vi "py.create.Pitch.vi"(8 "error in (no error)":errorcluster, 11 "Parameters":variant) -> (0 "error out":errorcluster, 3 "bytes":u8[](array[numeric]) format="%.0x")   [LabVIEW 2020]
uses:
  AddOrder/AddOrderLong.Parameters.ctl
  Time/Time.Parameters.ctl
  OrderExecuted/OrderExecuted.Parameters.ctl
  ReduceSize/ReduceSizeLong.Parameters.ctl
  ReduceSize/ReduceSizeShort.Parameters.ctl
  ModifyOrder/ModifyOrderLong.Parameters.ctl
  ModifyOrder/ModifyOrderShort.Parameters.ctl
  DeleteOrder/DeleteOrder.Parameters.ctl
  Trade/TradeLong.Parameters.ctl
  Trade/TradeShort.Parameters.ctl
  Trade/TradeExpanded.Parameters.ctl
  AddOrder/AddOrderShort.Parameters.ctl
  AddOrder/AddOrderExpanded.Parameters.ctl
  OrderExecuted/OrderExecutedAtPriceSize.Parameters.ctl
  <vilib>/Utility/Data Type/NI_Data Type.lvlib
  AddOrder/AddOrderLong.lvclass
  Time/Time.lvclass
  OrderExecuted/OrderExecuted.lvclass
  ReduceSize/ReduceSizeLong.lvclass
  ReduceSize/ReduceSizeShort.lvclass
  ModifyOrder/ModifyOrderLong.lvclass
  ModifyOrder/ModifyOrderShort.lvclass
  DeleteOrder/DeleteOrder.lvclass
  Trade/TradeLong.lvclass
  Trade/TradeShort.lvclass
  Trade/TradeExpanded.lvclass
  AddOrder/AddOrderShort.lvclass
  AddOrder/AddOrderExpanded.lvclass
  OrderExecuted/OrderExecutedAtPriceSize.lvclass
panel:
  out "return value":string
  out "Application Directory":path
  out "name":string
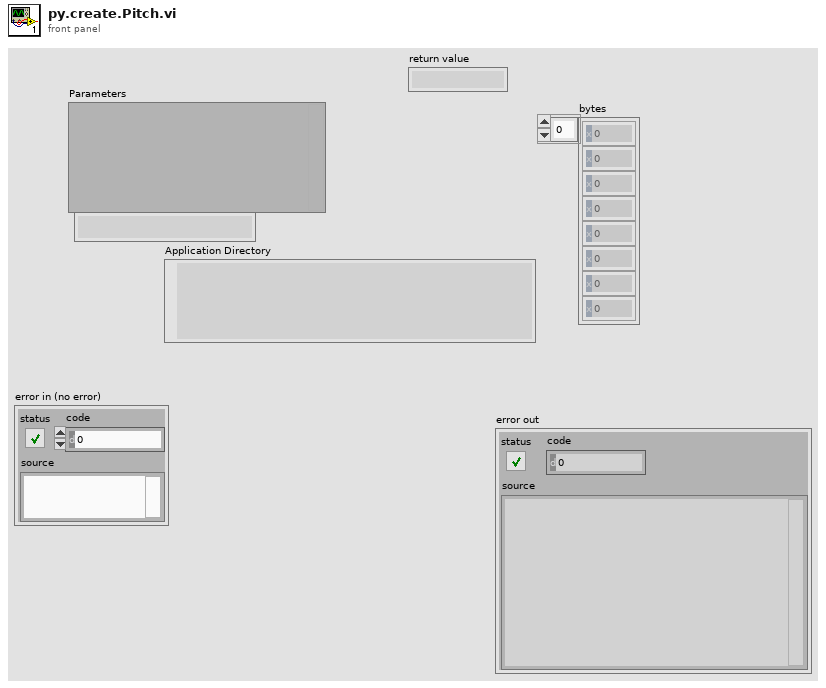
[diagram p1: front panel]
types:
  T1 = typedef "AddOrderLong.lvclass/AddOrderLong.Parameters.ctl" = cluster{"Time Offset":u32, "Order Id":string, "Quantity":u32, "Symbol":string, "Side Indicator":string, "Price":dbl}
  T2 = typedef "Time.lvclass/Time.Parameters.ctl" = cluster{"Time":u32}
  T3 = typedef "OrderExecuted.lvclass/OrderExecuted.Parameters.ctl" = cluster{"Time Offset":u32, "Order Id":string, "Executed Quantity":u32, "Execution Id":string}
  T4 = typedef "ReduceSizeLong.lvclass/ReduceSizeLong.Parameters.ctl" = cluster{"Time Offset":u32, "Order Id":string, "Canceled Quantity":u32}
  T5 = typedef "ReduceSizeShort.lvclass/ReduceSizeShort.Parameters.ctl" = cluster{"Time Offset":u32, "Order Id":string, "Canceled Quantity":u16}
  T6 = typedef "ModifyOrderLong.lvclass/ModifyOrderLong.Parameters.ctl" = cluster{"Time Offset":u32, "Order Id":string, "Quantity":u32, "Price":dbl, "Modify Flags":u8}
  T7 = typedef "ModifyOrderShort.lvclass/ModifyOrderShort.Parameters.ctl" = cluster{"Time Offset":u32, "Order Id":string, "Quantity":u32, "Price":u16, "Modify Flags":u8}
  T8 = typedef "DeleteOrder.lvclass/DeleteOrder.Parameters.ctl" = cluster{"Time Offset":u32, "Order Id":string}
  T9 = typedef "TradeLong.lvclass/TradeLong.Parameters.ctl" = cluster{"Time Offset":u32, "Order Id":string, "Execution Id":string, "Quantity":u32, "Price":dbl, "Side Indicator":string, "Symbol":string}
  T10 = typedef "TradeShort.lvclass/TradeShort.Parameters.ctl" = cluster{"Time Offset":u32, "Order Id":string, "Execution Id":string, "Quantity":u32, "Price":dbl, "Side Indicator":string, "Symbol":string}
  T11 = typedef "TradeExpanded.lvclass/TradeExpanded.Parameters.ctl" = cluster{"Time Offset":u32, "Order Id":string, "Side Indicator":string, "Quantity":u32, "Symbol":string, "Price":dbl, "Execution Id":string}
  T12 = typedef "AddOrderShort.lvclass/AddOrderShort.Parameters.ctl" = cluster{"Time Offset":u32, "Order Id":string, "Quantity":u32, "Symbol":string, "Side Indicator":string, "Price":dbl}
  T13 = typedef "AddOrderExpanded.lvclass/AddOrderExpanded.Parameters.ctl" = cluster{"Time Offset":u32, "Order Id":string, "Quantity":u32, "Symbol":string, "Side Indicator":string, "Price":dbl, "Participant Id":string, "Customer Indicator":string}
  T14 = typedef "OrderExecutedAtPriceSize.lvclass/OrderExecutedAtPriceSize.Parameters.ctl" = cluster{"Time Offset":u32, "Order Id":string, "Executed Quantity":u32, "Execution Id":string, "Remaining Quantity":u32, "Price":dbl}
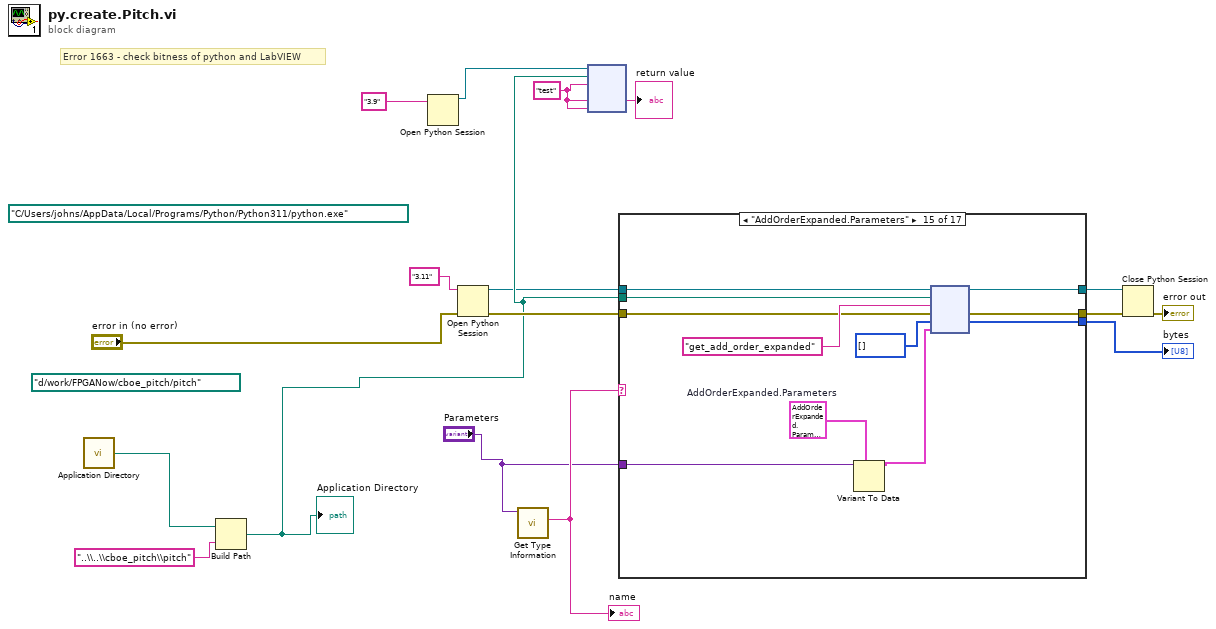
[diagram p0: block diagram]
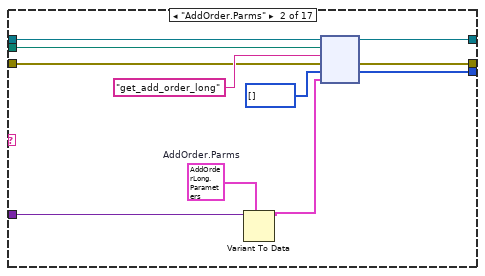
[diagram p3: hidden frame]
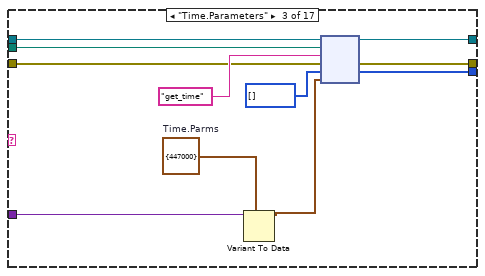
[diagram p4: hidden frame]
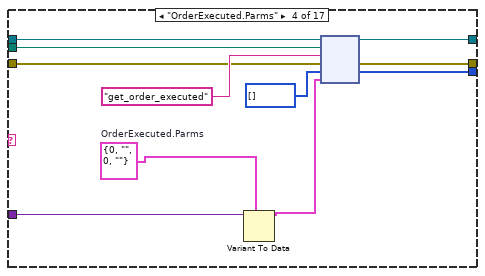
[diagram p5: hidden frame]
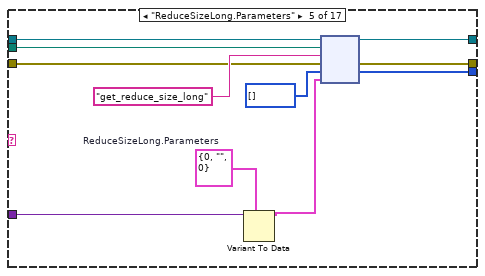
[diagram p6: hidden frame]
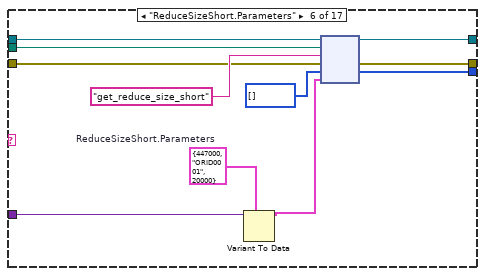
[diagram p7: hidden frame]
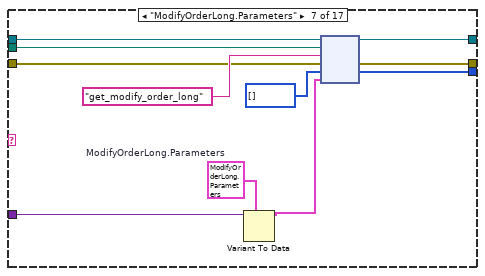
[diagram p8: hidden frame]
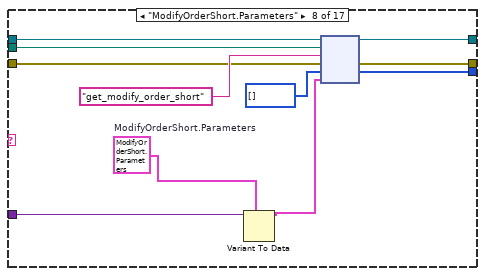
[diagram p9: hidden frame]
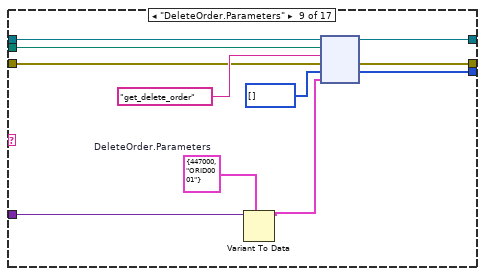
[diagram p10: hidden frame]
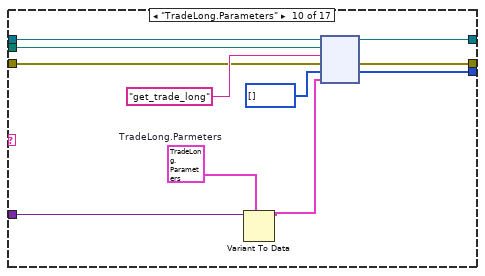
[diagram p11: hidden frame]
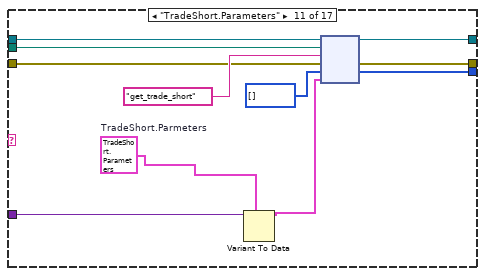
[diagram p12: hidden frame]
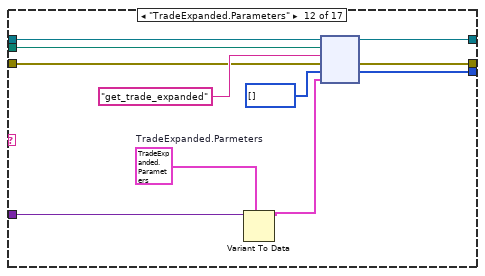
[diagram p13: hidden frame]
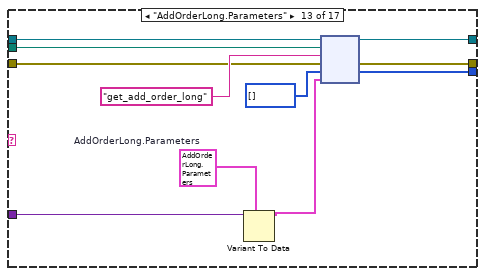
[diagram p14: hidden frame]
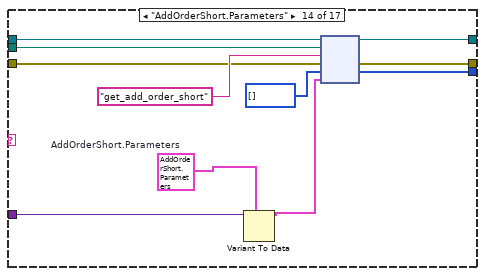
[diagram p15: hidden frame]
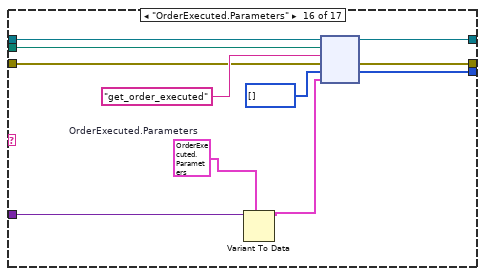
[diagram p16: hidden frame]
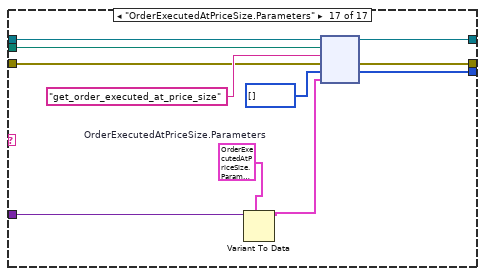
[diagram p17: hidden frame]
diagram:
  w3 = "test" ("function name")
  (unwired) path "C:/Users/johns/AppData/Local/Programs/Python/Python311/python.exe" ("Python path")
  (unwired) path "d:/work/FPGANow/cboe_pitch/pitch" ("module path")
  # "Error 1663 - check bitness of python and LabVIEW"
  n1 = call <vilib>:"Application Directory.vi"() -> ("Application Directory"=w8:path)
  n2 = Build Path(base path=w8, name or relative path="..\\..\\cboe_pitch\\pitch") -> (appended path=w6:path)
  "Application Directory" <- w6
  n3 = Open Python Session(python version="3.9" ("Python version")) -> (session out=w1:refnum<k35>)  [unwired: 2 in, 1 out]
  n4 = Open Python Session(python version="3.11" ("Python version"), 3:"error in (no error)") -> (session out=w5:refnum<k35>, error out=w14:errorcluster)  [unwired: 1 in]
  n5 = call <vilib>:"Get Type Information.vi"("variant"="Parameters") -> ("name"=w10:string)  [unwired: 6 in, 4 out]
  "name" <- w10
  n6 = node(w1, w6, w3, w3, w3) -> (→"return value":string)  [unwired: 2 in, 4 out]
  n7 = case shown="\"AddOrderExpanded.Parameters\"" w10 {
    tunnel: w5 -> [w19 w30 w41 w52 w63 w74 w85 w96 w107 w118 w129 w140 w151 w162 w173 w184 w195]
    tunnel: [w19 w29 w40 w51 w62 w73 w84 w95 w106 w117 w128 w139 w150 w161 w172 w183 w194] -> w17
    tunnel: w6 -> [_ w28 w39 w50 w61 w72 w83 w94 w105 w116 w127 w138 w149 w160 w171 w182 w193]
    tunnel: [w18 w27 w38 w49 w60 w71 w82 w93 w104 w115 w126 w137 w148 w159 w170 w181 w192] -> w15
    tunnel: w14 -> [w18 w25 w36 w47 w58 w69 w80 w91 w102 w113 w124 w135 w146 w157 w168 w179 w190]
    tunnel: [_ w24 w35 w46 w57 w68 w79 w90 w101 w112 w123 w134 w145 w156 w167 w178 w189] -> w13
    tunnel: "Parameters" -> [_ w22 w33 w44 w55 w66 w77 w88 w99 w110 w121 w132 w143 w154 w165 w176 w187]
    frame "False", Default {
    }
    frame "AddOrder.Parms" {
      w21 = T1 {"Time Offset"=447000, "Order Id"="ORID0001", "Quantity"=20000, "Symbol"="AAPL", "Side Indicator"="B", "Price"=0.905}  # AddOrder.Parms
      n8 = Variant To Data(type=w21, Variant=w22) -> (data=w20:T1)  [unwired: 1 in, 1 out]
      n9 = node(w30, w28, "get_add_order_long" ("function name"), w25, u8[] [], w20) -> (w29:refnum<k35>, w27:errorcluster, w24:u8[])  [unwired: 1 in, 2 out]
    }
    frame "Time.Parameters" {
      w31 = T2 {"Time"=447000}  # Time.Parms
      n10 = Variant To Data(type=w31, Variant=w33) -> (data=w32:T2)  [unwired: 1 in, 1 out]
      n11 = node(w41, w39, "get_time" ("function name"), w36, u8[] [], w32) -> (w40:refnum<k35>, w38:errorcluster, w35:u8[])  [unwired: 1 in, 2 out]
    }
    frame "OrderExecuted.Parms" {
      w42 = T3 {"Time Offset"=0, "Order Id"="", "Executed Quantity"=0, "Execution Id"=""}  # OrderExecuted.Parms
      n12 = Variant To Data(type=w42, Variant=w44) -> (data=w43:T3)  [unwired: 1 in, 1 out]
      n13 = node(w52, w50, "get_order_executed" ("function name"), w47, u8[] [], w43) -> (w51:refnum<k35>, w49:errorcluster, w46:u8[])  [unwired: 1 in, 2 out]
    }
    frame "ReduceSizeLong.Parameters" {
      w53 = T4 {"Time Offset"=0, "Order Id"="", "Canceled Quantity"=0}  # ReduceSizeLong.Parameters
      n14 = Variant To Data(type=w53, Variant=w55) -> (data=w54:T4)  [unwired: 1 in, 1 out]
      n15 = node(w63, w61, "get_reduce_size_long" ("function name"), w58, u8[] [], w54) -> (w62:refnum<k35>, w60:errorcluster, w57:u8[])  [unwired: 1 in, 2 out]
    }
    frame "ReduceSizeShort.Parameters" {
      w64 = T5 {"Time Offset"=447000, "Order Id"="ORID0001", "Canceled Quantity"=20000}  # ReduceSizeShort.Parameters
      n16 = Variant To Data(type=w64, Variant=w66) -> (data=w65:T5)  [unwired: 1 in, 1 out]
      n17 = node(w74, w72, "get_reduce_size_short" ("function name"), w69, u8[] [], w65) -> (w73:refnum<k35>, w71:errorcluster, w68:u8[])  [unwired: 1 in, 2 out]
    }
    frame "ModifyOrderLong.Parameters" {
      w75 = T6 {"Time Offset"=447000, "Order Id"="ORID0001", "Quantity"=20000, "Price"=0.905, "Modify Flags"=1}  # ModifyOrderLong.Parameters
      n18 = Variant To Data(type=w75, Variant=w77) -> (data=w76:T6)  [unwired: 1 in, 1 out]
      n19 = node(w85, w83, "get_modify_order_long" ("function name"), w80, u8[] [], w76) -> (w84:refnum<k35>, w82:errorcluster, w79:u8[])  [unwired: 1 in, 2 out]
    }
    frame "ModifyOrderShort.Parameters" {
      w86 = T7 {"Time Offset"=447000, "Order Id"="ORID0001", "Quantity"=20000, "Price"=1, "Modify Flags"=1}  # ModifyOrderShort.Parameters
      n20 = Variant To Data(type=w86, Variant=w88) -> (data=w87:T7)  [unwired: 1 in, 1 out]
      n21 = node(w96, w94, "get_modify_order_short" ("function name"), w91, u8[] [], w87) -> (w95:refnum<k35>, w93:errorcluster, w90:u8[])  [unwired: 1 in, 2 out]
    }
    frame "DeleteOrder.Parameters" {
      w97 = T8 {"Time Offset"=447000, "Order Id"="ORID0001"}  # DeleteOrder.Parameters
      n22 = Variant To Data(type=w97, Variant=w99) -> (data=w98:T8)  [unwired: 1 in, 1 out]
      n23 = node(w107, w105, "get_delete_order" ("function name"), w102, u8[] [], w98) -> (w106:refnum<k35>, w104:errorcluster, w101:u8[])  [unwired: 1 in, 2 out]
    }
    frame "TradeLong.Parameters" {
      w108 = T9 {"Time Offset"=447000, "Order Id"="ORID0001", "Execution Id"="EXE_ID_1", "Quantity"=20000, "Price"=0.905, "Side Indicator"="B", "Symbol"="AAPL"}  # TradeLong.Parmeters
      n24 = Variant To Data(type=w108, Variant=w110) -> (data=w109:T9)  [unwired: 1 in, 1 out]
      n25 = node(w118, w116, "get_trade_long" ("function name"), w113, u8[] [], w109) -> (w117:refnum<k35>, w115:errorcluster, w112:u8[])  [unwired: 1 in, 2 out]
    }
    frame "TradeShort.Parameters" {
      w119 = T10 {"Time Offset"=447000, "Order Id"="ORID0001", "Execution Id"="EXE_ID_1", "Quantity"=20000, "Price"=0.905, "Side Indicator"="B", "Symbol"="AAPL"}  # TradeShort.Parmeters
      n26 = Variant To Data(type=w119, Variant=w121) -> (data=w120:T10)  [unwired: 1 in, 1 out]
      n27 = node(w129, w127, "get_trade_short" ("function name"), w124, u8[] [], w120) -> (w128:refnum<k35>, w126:errorcluster, w123:u8[])  [unwired: 1 in, 2 out]
    }
    frame "TradeExpanded.Parameters" {
      w130 = T11 {"Time Offset"=447000, "Order Id"="ORID0001", "Side Indicator"="B", "Quantity"=20000, "Symbol"="AAPL", "Price"=0.905, "Execution Id"="EXE_ID_1"}  # TradeExpanded.Parmeters
      n28 = Variant To Data(type=w130, Variant=w132) -> (data=w131:T11)  [unwired: 1 in, 1 out]
      n29 = node(w140, w138, "get_trade_expanded" ("function name"), w135, u8[] [], w131) -> (w139:refnum<k35>, w137:errorcluster, w134:u8[])  [unwired: 1 in, 2 out]
    }
    frame "AddOrderLong.Parameters" {
      w141 = T1 {"Time Offset"=447000, "Order Id"="ORID0001", "Quantity"=20000, "Symbol"="AAPL", "Side Indicator"="B", "Price"=0.905}  # AddOrderLong.Parameters
      n30 = Variant To Data(type=w141, Variant=w143) -> (data=w142:T1)  [unwired: 1 in, 1 out]
      n31 = node(w151, w149, "get_add_order_long" ("function name"), w146, u8[] [], w142) -> (w150:refnum<k35>, w148:errorcluster, w145:u8[])  [unwired: 1 in, 2 out]
    }
    frame "AddOrderShort.Parameters" {
      w152 = T12 {"Time Offset"=447000, "Order Id"="ORID0001", "Quantity"=20000, "Symbol"="AAPL", "Side Indicator"="B", "Price"=0.905}  # AddOrderShort.Parameters
      n32 = Variant To Data(type=w152, Variant=w154) -> (data=w153:T12)  [unwired: 1 in, 1 out]
      n33 = node(w162, w160, "get_add_order_short" ("function name"), w157, u8[] [], w153) -> (w161:refnum<k35>, w159:errorcluster, w156:u8[])  [unwired: 1 in, 2 out]
    }
    frame "AddOrderExpanded.Parameters" {
      w163 = T13 {"Time Offset"=447000, "Order Id"="ORID0001", "Quantity"=20000, "Symbol"="AAPL", "Side Indicator"="B", "Price"=0.905, "Participant Id"="B", "Customer Indicator"="B"}  # AddOrderExpanded.Parameters
      n34 = Variant To Data(type=w163, Variant=w165) -> (data=w164:T13)  [unwired: 1 in, 1 out]
      n35 = node(w173, w171, "get_add_order_expanded" ("function name"), w168, u8[] [], w164) -> (w172:refnum<k35>, w170:errorcluster, w167:u8[])  [unwired: 1 in, 2 out]
    }
    frame "OrderExecuted.Parameters" {
      w174 = T3 {"Time Offset"=447000, "Order Id"="ORID0001", "Executed Quantity"=20000, "Execution Id"="AAPL"}  # OrderExecuted.Parameters
      n36 = Variant To Data(type=w174, Variant=w176) -> (data=w175:T3)  [unwired: 1 in, 1 out]
      n37 = node(w184, w182, "get_order_executed" ("function name"), w179, u8[] [], w175) -> (w183:refnum<k35>, w181:errorcluster, w178:u8[])  [unwired: 1 in, 2 out]
    }
    frame "OrderExecutedAtPriceSize.Parameters" {
      w185 = T14 {"Time Offset"=447000, "Order Id"="ORID0001", "Executed Quantity"=20000, "Execution Id"="AAPL", "Remaining Quantity"=20000, "Price"=0.905}  # OrderExecutedAtPriceSize.Parameters
      n38 = Variant To Data(type=w185, Variant=w187) -> (data=w186:T14)  [unwired: 1 in, 1 out]
      n39 = node(w195, w193, "get_order_executed_at_price_size" ("function name"), w190, u8[] [], w186) -> (w194:refnum<k35>, w192:errorcluster, w189:u8[])  [unwired: 1 in, 2 out]
    }
  }
  "bytes" <- w13
  n40 = Close Python Session(session in=w17, error in=w15) -> (11:→"error out":errorcluster)
